vi "CRYIntermodulation Freq Calc.vi"(0 "Type":u16, 5 "Freq1 In":dbl, 7 "Freq2 In":dbl, 9 "Orders":dbl[](array[numeric]), 11 "Fs":dbl) -> (4 "Frequency Array Out":dbl[](array[numeric]))   [LabVIEW 2013]
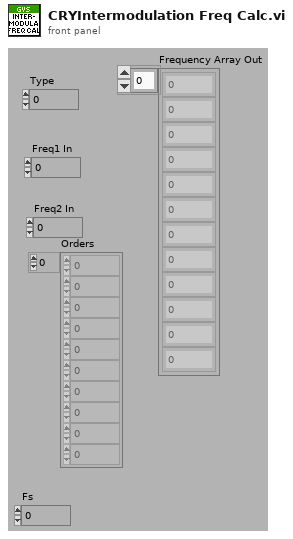
[diagram p1: front panel]
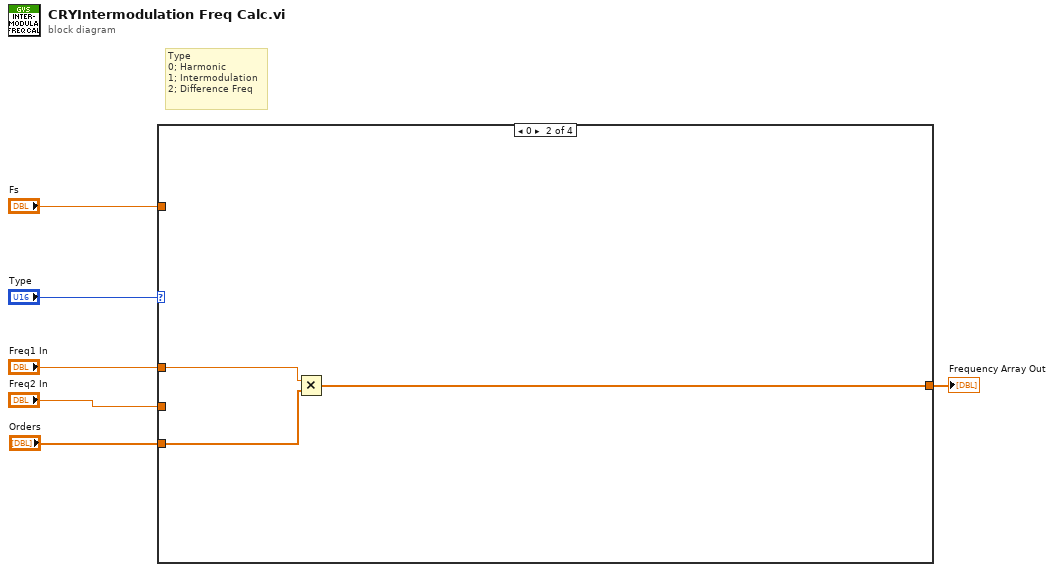
[diagram p0: block diagram]
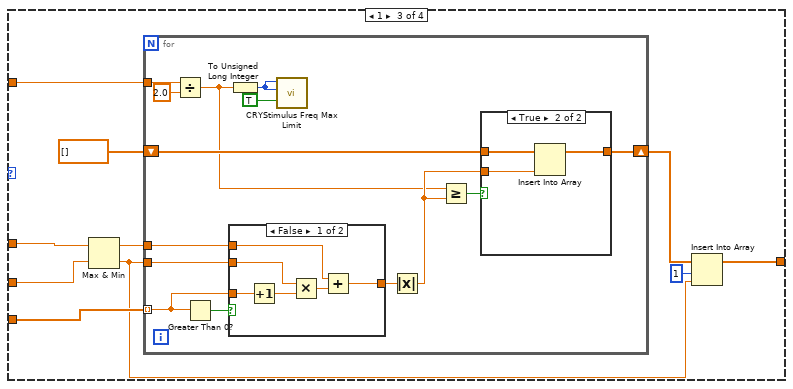
[diagram p3: hidden frame]
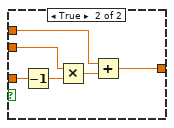
[diagram p5: hidden frame]
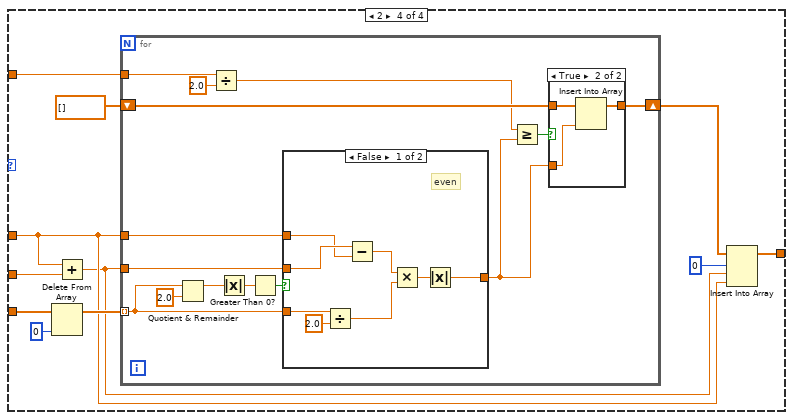
[diagram p6: hidden frame]
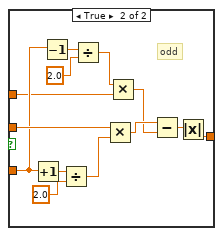
[diagram p8: hidden frame]
diagram:
  # "Type\n0; Harmonic\n1; Intermodulation\n2; Difference Freq"
  n1 = case shown="0" "Type" {
    tunnel: "Orders" -> [_ w8 w19 w60]
    tunnel: "Freq1 In" -> [_ w9 w18 w52]
    tunnel: "Freq2 In" -> [_ _ w17 w51]
    tunnel: [_ w7 w12 w54] -> w2
    tunnel: "Fs" -> [_ _ w15 w56]
    frame Default {
    }
    frame 0 {
      n2 = Multiply(x=w9, y=w8) -> (x*y=w7:dbl[])
    }
    frame 1 {
      n3 = Max & Min(x=w18, y=w17) -> (max(x,y)=w16:dbl, min(x,y)=w10:dbl)
      n4 = for {
        tunnel: w16 -> [w32]
        tunnel: w10 -> [w31]
        tunnel: w19 -> [w30] mode=indexing
        shift-right: [w25] -> w13
        shift-left: dbl[] [] ("Orders") -> [w27]
        tunnel: w15 -> [w21]
        n5 = Divide(x=w21, y=2.0) -> (x/y=w20:dbl)
        n6 = Greater Than 0?(x=w30) -> (x > 0?=w33:bool)
        n7 = case shown="False" w33 {
          tunnel: w32 -> [w40 w46]
          tunnel: w31 -> [w42 w47]
          tunnel: w30 -> [w43 w49]
          tunnel: [w38 w44] -> w29
          frame False {
            n8 = Increment(x=w43) -> (x+1=w41:dbl)
            n9 = Multiply(x=w42, y=w41) -> (x*y=w39:dbl)
            n10 = Add(x=w40, y=w39) -> (x+y=w38:dbl)
          }
          frame True {
            n11 = Decrement(x=w49) -> (x-1=w48:dbl)
            n12 = Multiply(x=w47, y=w48) -> (x*y=w45:dbl)
            n13 = Add(x=w46, y=w45) -> (x+y=w44:dbl)
          }
        }
        n14 = To Unsigned Long Integer(number=w20) -> (unsigned 32bit integer=w23:u32)
        n15 = call "CRYStimulus Freq Max Limit.vi"("Decrement Flag"=TRUE, "Max Freq"=w23, "Input Val"=w23) -> ()  [unwired: 1 in, 8 out]
        n16 = Absolute Value(x=w29) -> (abs(x)=w26:dbl)
        n17 = Greater Or Equal?(x=w20, y=w26) -> (x >= y?=w28:bool)
        n18 = case shown="True" w28 {
          tunnel: w27 -> [w34 w37]
          tunnel: w26 -> [_ w36]
          tunnel: [w34 w35] -> w25
          frame False {
          }
          frame True {
            n19 = Insert Into Array(array=w37, new element=w36) -> (w35:dbl[])  [unwired: 1 in]
          }
        }
      }
      n20 = Insert Into Array(array=w13, index=1, new element=w10) -> (w12:dbl[])
    }
    frame 2 {
      n21 = Delete From Array(array=w60, index=0) -> (array with subset deleted=w59:dbl[])  [unwired: 1 in, 1 out]
      n22 = Add(x=w52, y=w51) -> (x+y=w50:dbl)
      n23 = for {
        tunnel: w59 -> [w66] mode=indexing
        tunnel: w52 -> [w74]
        tunnel: w50 -> [w73]
        shift-right: [w69] -> w55
        shift-left: dbl[] [] ("Orders") -> [w70]
        tunnel: w56 -> [w62]
        n24 = Quotient & Remainder(x=w66, y=2.0) -> (x-y*floor(x/y)=w64:dbl)  [unwired: 1 out]
        n25 = Divide(x=w62, y=2.0) -> (x/y=w61:dbl)
        n26 = Absolute Value(x=w64) -> (abs(x)=w72:dbl)
        n27 = Greater Than 0?(x=w72) -> (x > 0?=w71:bool)
        n28 = case shown="False" w71 {
          tunnel: w66 -> [w86 w95]
          tunnel: w74 -> [w83 w92]
          tunnel: w73 -> [w84 w97]
          tunnel: [w79 w87] -> w68
          frame False {
            # "even"
            n29 = Divide(x=w86, y=2.0) -> (x/y=w81:dbl)
            n30 = Subtract(x=w84, y=w83) -> (x-y=w82:dbl)
            n31 = Multiply(x=w82, y=w81) -> (x*y=w80:dbl)
            n32 = Absolute Value(x=w80) -> (abs(x)=w79:dbl)
          }
          frame True {
            # "odd"
            n33 = Increment(x=w95) -> (x+1=w99:dbl)
            n34 = Decrement(x=w95) -> (x-1=w94:dbl)
            n35 = Divide(x=w99, y=2.0) -> (x/y=w96:dbl)
            n36 = Divide(x=w94, y=2.0) -> (x/y=w91:dbl)
            n37 = Multiply(x=w97, y=w96) -> (x*y=w90:dbl)
            n38 = Multiply(x=w91, y=w92) -> (x*y=w89:dbl)
            n39 = Subtract(x=w90, y=w89) -> (x-y=w88:dbl)
            n40 = Absolute Value(x=w88) -> (abs(x)=w87:dbl)
          }
        }
        n41 = Greater Or Equal?(x=w61, y=w68) -> (x >= y?=w67:bool)
        n42 = case shown="True" w67 {
          tunnel: w70 -> [w75 w78]
          tunnel: w68 -> [_ w77]
          tunnel: [w75 w76] -> w69
          frame False {
          }
          frame True {
            n43 = Insert Into Array(array=w78, new element=w77) -> (w76:dbl[])  [unwired: 1 in]
          }
        }
      }
      n44 = Insert Into Array(array=w55, index=0, new element #1=w50, new element #2=w52) -> (w54:dbl[])
    }
  }
  "Frequency Array Out" <- w2
